vi "Update Ballard Status Error Count.vi"(9 "status error counts":T1, 10 "values in":dbl[](array[numeric]), 11 "Rx execution unit in":refnum<class "Rx Execution Unit.lvclass">) -> (2 "values out":dbl[](array[numeric]), 3 "Rx execution unit out":refnum<class "Rx Execution Unit.lvclass">)   [LabVIEW 2020, in "AIM MIL-STD-1553 Engine.lvlib" / "Implementation.lvlib" / "Rx Execution Unit.lvclass"]
uses:
  Rx Execution Unit.lvclass
  Status Error Counts.ctl
  Rx Execution Unit.lvclass/Rx Execution Unit.ctl
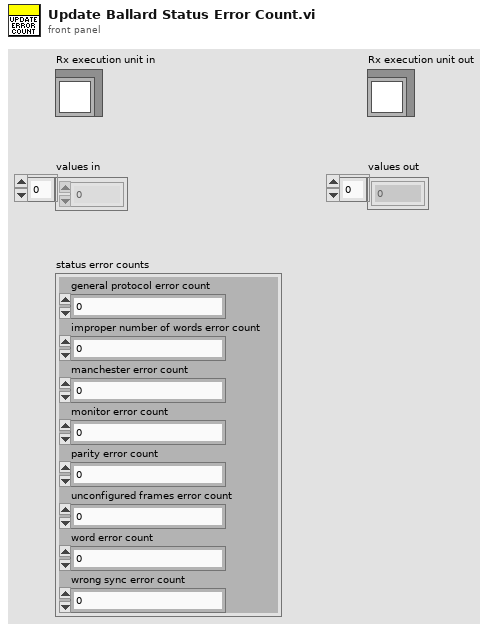
[diagram p1: front panel]
types:
  T1 = typedef "AIM MIL-STD-1553 Engine.lvlib/Implementation.lvlib/Rx Execution Unit.lvclass/Status Error Counts.ctl" = cluster{"general protocol error count":u64, "improper number of words error count":u64, "manchester error count":u64, "monitor error count":u64, "parity error count":u64, "unconfigured frames error count":u64, "word error count":u64, "wrong sync error count":u64}
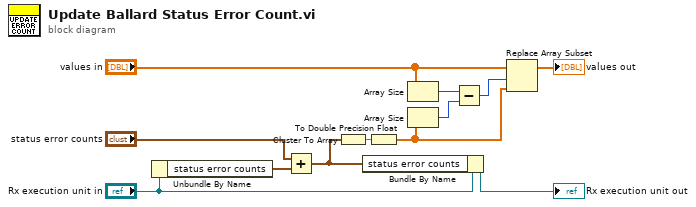
[diagram p0: block diagram]
diagram:
  n1 = Unbundle By Name("Rx execution unit in") -> ("status error counts"=w5:T1)
  n2 = Add(x="status error counts", y=w5) -> (x+y=w3:T1)
  n3 = Cluster To Array(cluster=w3) -> (array=w2:u64[])
  n4 = Bundle By Name(cluster="Rx execution unit in", "status error counts"=w3) -> (→"Rx execution unit out":refnum<class "Rx Execution Unit.lvclass">)
  n5 = To Double Precision Float(number=w2) -> (double precision float=w1:dbl[])
  n6 = Array Size(array="values in") -> (size(s)=w10:i32)
  n7 = Array Size(array=w1) -> (size(s)=w9:i32)
  n8 = Subtract(x=w10, y=w9) -> (x-y=w7:i32)
  n9 = Replace Array Subset(array="values in", new element=w1, index=w7) -> (→"values out":dbl[])
